vi "Operator judge LVDT's TVS.vi"(6 "LVDT's Limits":T1[](array[typedef]) {"Lower Limit" format="%.2f"; "Upper Limit" format="%.2f"}, 11 "LVDT's Array":sgl[](array[numeric])) -> ()   [LabVIEW 2018]
uses:
  type defs/EOL LVDT's Check Controller.ctl
panel:
  out "E3":dbl(slide) min=-5.0 max=5.0 scale=-5.0..5.0 scale format="%#_4g"
  out "E4":dbl(slide) min=-5.0 max=5.0 scale=-5.0..5.0 scale format="%#_4g"
  out "E2":dbl(slide) min=-5.0 max=5.0 scale=-6.0..6.0 scale format="%#_4g"
  out "E1":dbl(slide) min=-5.0 max=5.0 scale=-5.0..5.0 scale format="%#_4g"
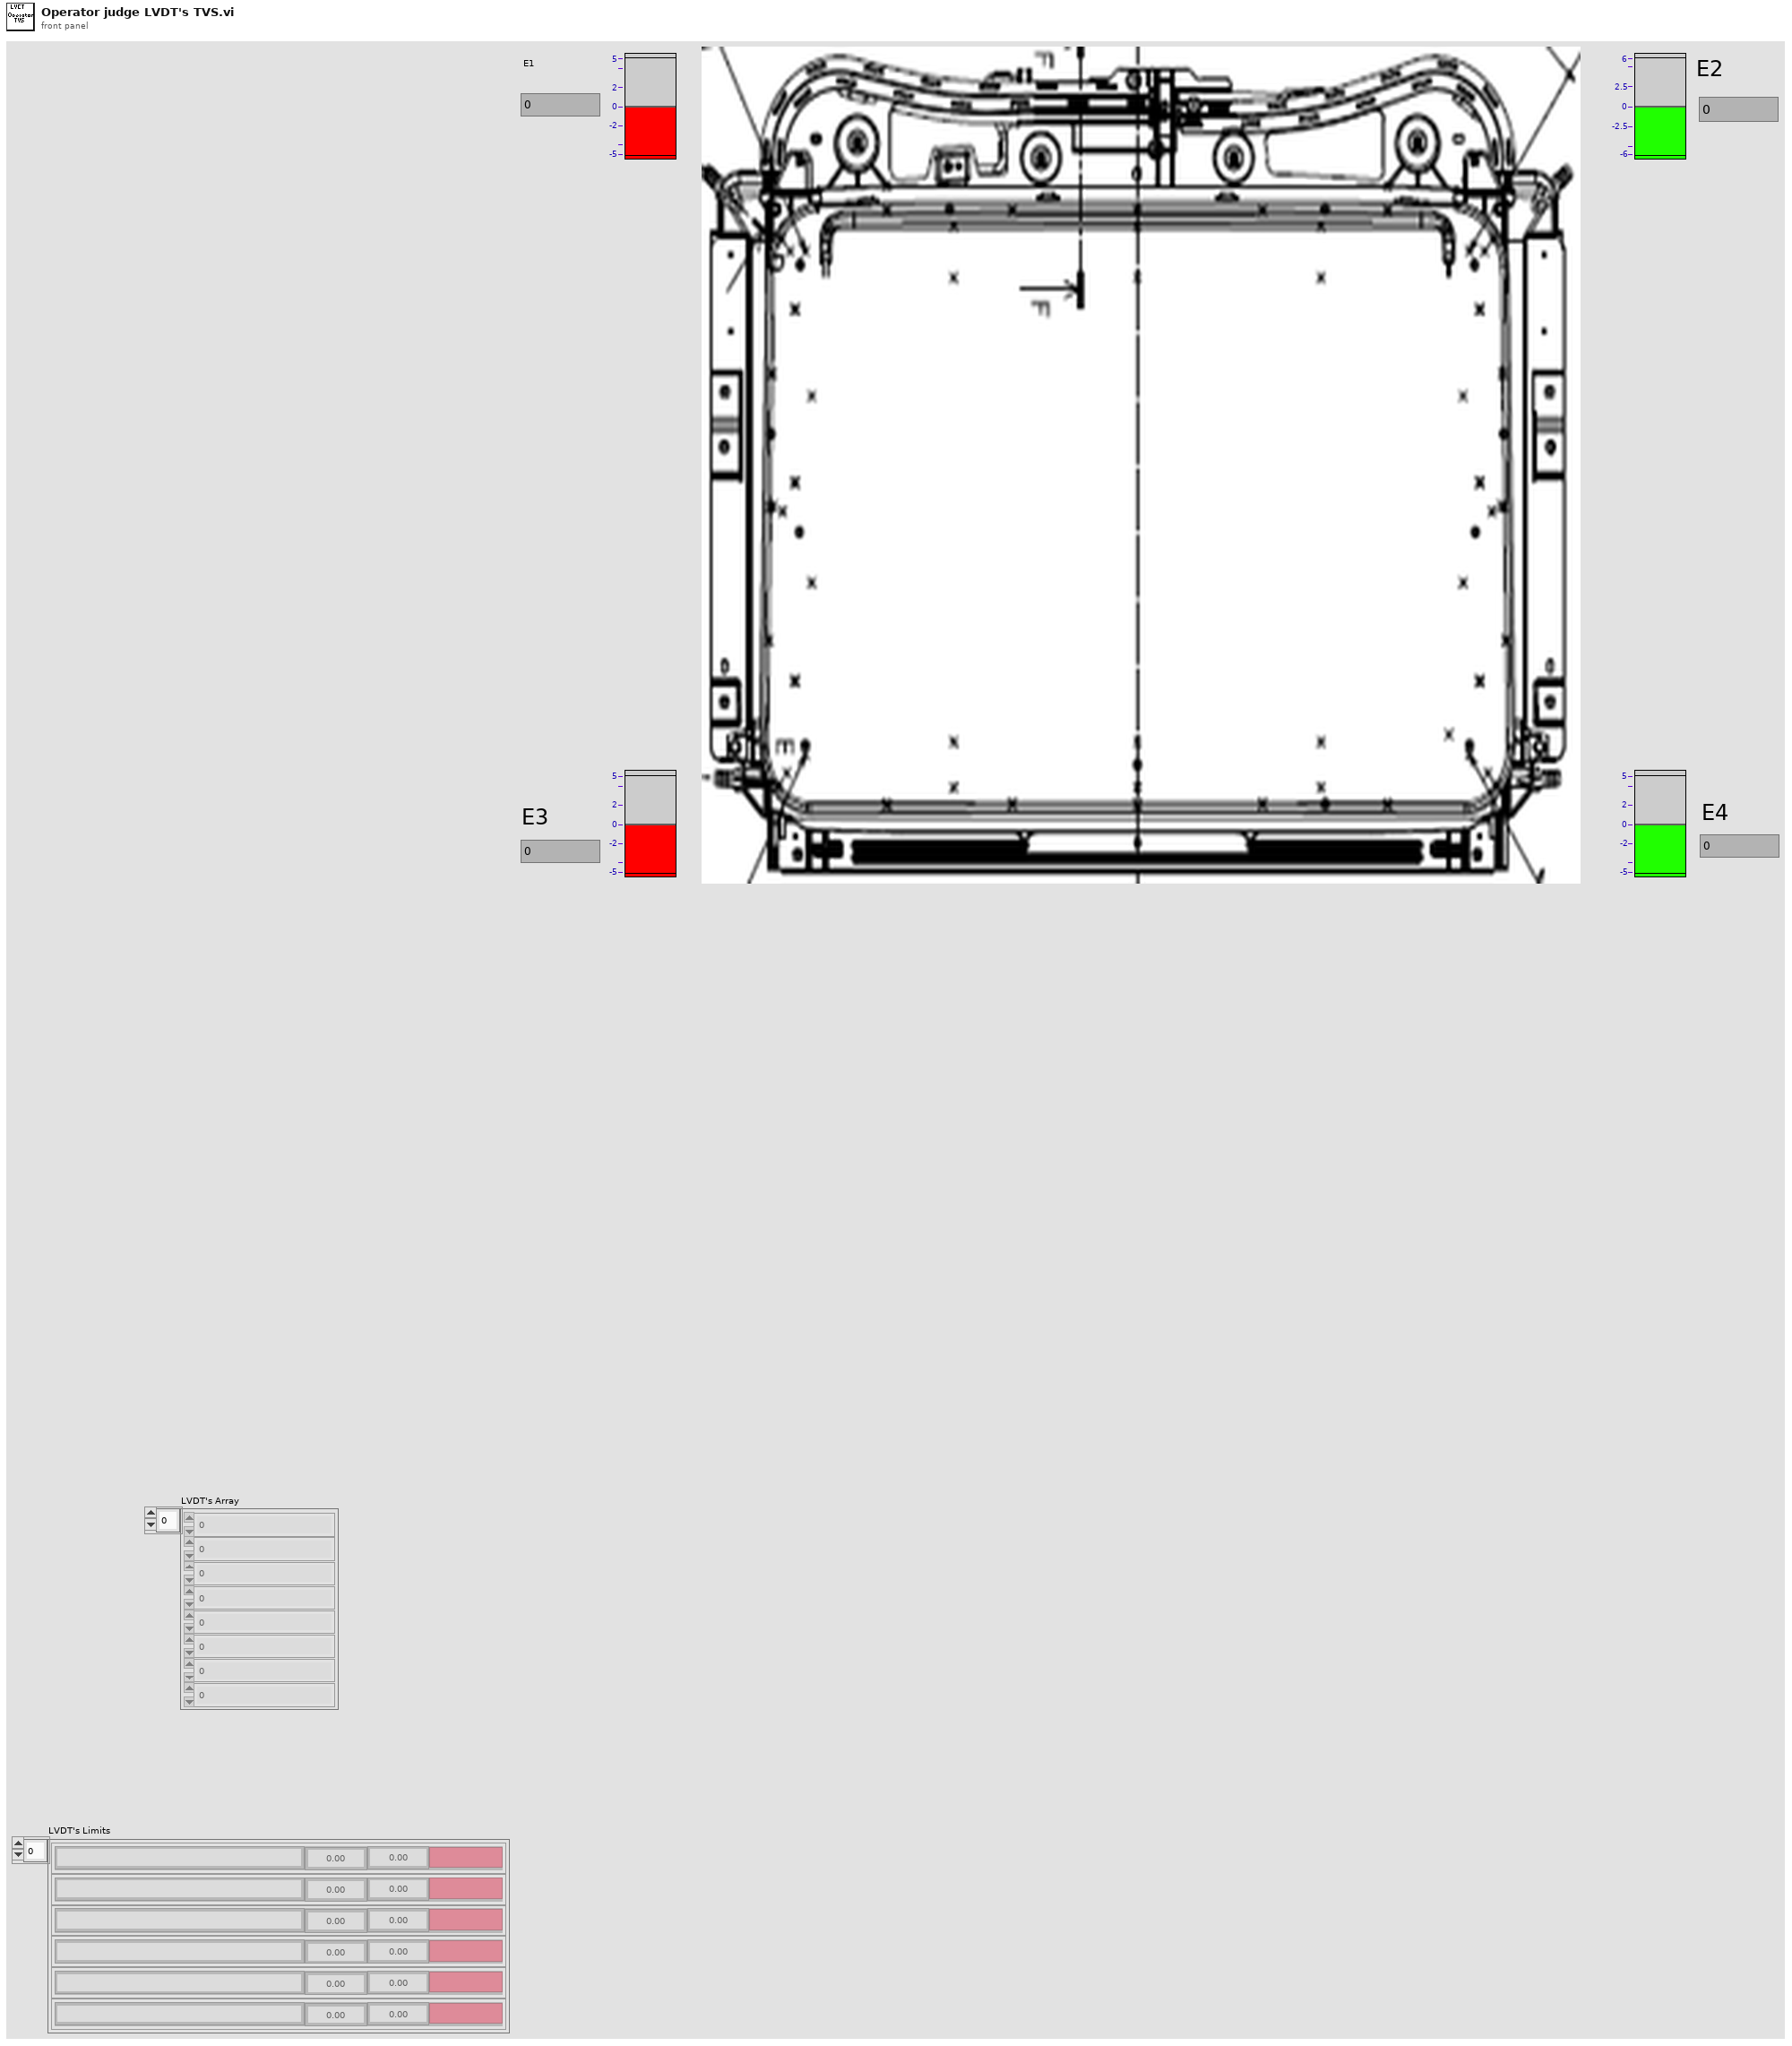
[diagram p1: front panel]
types:
  T1 = typedef "EOL LVDT's Check Controller.ctl" = cluster{"Upper Limit":dbl, "Lower Limit":dbl, "LVDT Name":string, "Check":bool}
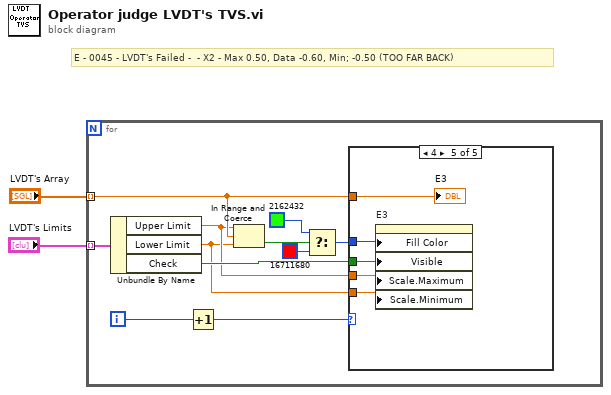
[diagram p0: block diagram]
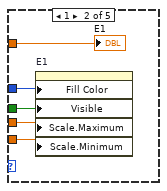
[diagram p3: hidden frame]
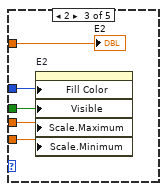
[diagram p4: hidden frame]
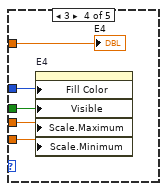
[diagram p5: hidden frame]
diagram:
  # "E - 0045 - LVDT's Failed -  - X2 - Max 0.50, Data -0.60, Min; -0.50 (TOO FAR BACK)"
  n1 = for {
    tunnel: "LVDT's Array" -> [w7] mode=indexing
    tunnel: "LVDT's Limits" -> [w13] mode=indexing
    i -> [w5]
    n2 = Unbundle By Name(w13) -> ("Upper Limit"=w4:dbl, "Lower Limit"=w3:dbl, "Check"=w12:bool)
    n3 = Increment(x=w5) -> (x+1=w6:i32)
    n4 = In Range and Coerce(upper limit=w4, x=w7, lower limit=w3) -> (In Range?=w9:bool)  [unwired: 1 out]
    n5 = Select(t=u32 2162432, s=w9, f=u32 16711680) -> (s? t:f=w8:u32)
    n6 = case shown="4" w6 {
      tunnel: w12 -> [_ w16 w21 w26 w31]
      tunnel: w8 -> [_ w17 w22 w27 w32]
      tunnel: w7 -> [_ w18 w23 w28 w33]
      tunnel: w4 -> [_ w15 w20 w25 w30]
      tunnel: w3 -> [_ w14 w19 w24 w29]
      frame 0, Default {
      }
      frame 1 {
        n7 = property on="E1" class="Slide (严格)"("Fill Color"=w17, "Visible"=w16, "Scale.Maximum"=w15, "Scale.Minimum"=w14) -> ()  [unwired: 2 in, 2 out]
        "E1" <- w18
      }
      frame 2 {
        n8 = property on="E2" class="Slide (严格)"("Fill Color"=w22, "Visible"=w21, "Scale.Maximum"=w20, "Scale.Minimum"=w19) -> ()  [unwired: 2 in, 2 out]
        "E2" <- w23
      }
      frame 3 {
        n9 = property on="E4" class="Slide (严格)"("Fill Color"=w27, "Visible"=w26, "Scale.Maximum"=w25, "Scale.Minimum"=w24) -> ()  [unwired: 2 in, 2 out]
        "E4" <- w28
      }
      frame 4 {
        n10 = property on="E3" class="Slide (严格)"("Fill Color"=w32, "Visible"=w31, "Scale.Maximum"=w30, "Scale.Minimum"=w29) -> ()  [unwired: 2 in, 2 out]
        "E3" <- w33
      }
    }
  }
